vi "Check for Valid File Paths.vi"(8 "error in (no error)":errorcluster, 11 "Input Paths Refnum":refnum<vi>) -> (0 "error out":errorcluster)   [LabVIEW 2014]
uses:
  Controls/Input Paths.ctl
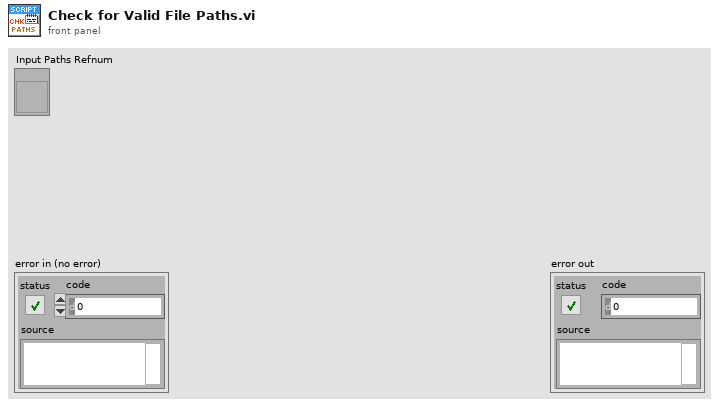
[diagram p1: front panel]
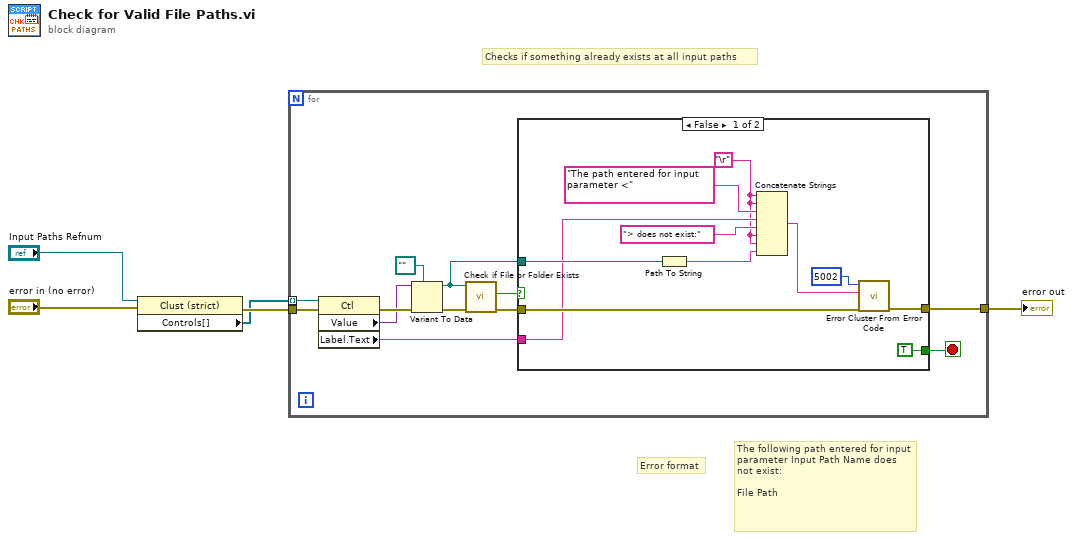
[diagram p0: block diagram]
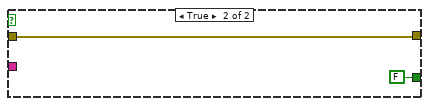
[diagram p2: hidden frame]
diagram:
  # "Error format"
  # "The following path entered for input parameter Input Path Name does not exist:\n\nFile Path"
  # "Checks if something already exists at all input paths"
  n1 = property class="Clust (strict)"(reference="Input Paths Refnum", error in="error in (no error)") -> (error out=w5:errorcluster, "Controls[]"=w4:refnum<vi>[])  [unwired: 1 out]
  n2 = for {
    tunnel: w5 -> [w17]
    tunnel: w4 -> [w16] mode=indexing
    tunnel: [w7] -> w2
    stop <- w6 stop-if-true
    n3 = property class="Ctl"(reference=w16, error in=w17) -> (error out=w15:errorcluster, "Value"=w12:variant, "Label.Text"=w9:string)  [unwired: 1 out]
    n4 = Variant To Data(error in=w15, type=path "", Variant=w12) -> (data=w8:path, error out=w14:errorcluster)
    n5 = call <vilib>:"Check if File or Folder Exists.vi"("error in (no error)"=w14, "path"=w8) -> ("error out"=w11:errorcluster, "file or folder exists?"=w10:bool)  [unwired: 7 in, 1 out]
    n6 = case shown="False" w10 {
      tunnel: w11 -> [w28 w30]
      tunnel: w9 -> [w21 _]
      tunnel: w8 -> [w25 _]
      tunnel: [w24 w30] -> w7
      tunnel: [TRUE FALSE] -> w6
      frame False {
        w18 = "\r"
        n7 = Path To String(path=w25) -> (string=w19:string)
        n8 = Concatenate Strings(w18, w18, "The path entered for input parameter <" ("string"), w21, "> does not exist:" ("string"), w18, w18, w19) -> (w27:string)
        n9 = call <vilib>:"Error Cluster From Error Code.vi"("error in (no error)"=w28, "error message (\"\")"=w27, "error code (0)"=5002) -> ("error out"=w24:errorcluster)  [unwired: 6 in]
      }
      frame True {
      }
    }
  }
  "error out" <- w2
